vi "Delete Recipe.vi"(8 "error in (no error)":errorcluster, 9 "Delete Row":u16, 11 "Masterv2 in":refnum<class "Masterv2.lvclass">) -> (0 "error out":errorcluster, 3 "Masterv2 out":refnum<class "Masterv2.lvclass">)   [LabVIEW 2014, in "Main Libraryv2.lvlib" / "Masterv2.lvclass"]
uses:
  Master/Masterv2.lvclass
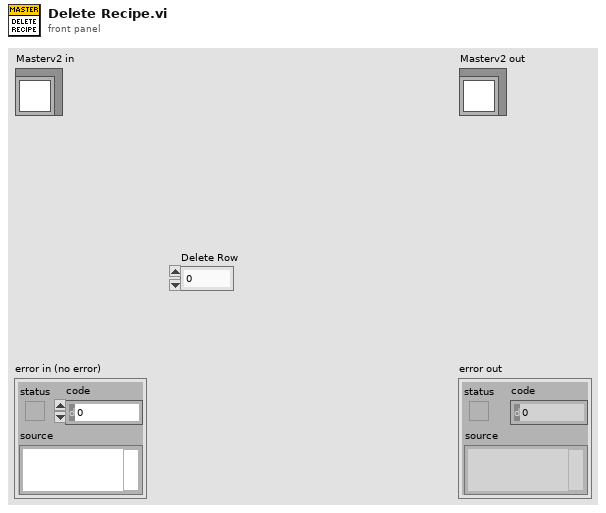
[diagram p1: front panel]
types:
  T1 = cluster{"Speed":string, "Temperature SP":string, "Time Limit":string, "Direction":string}[]
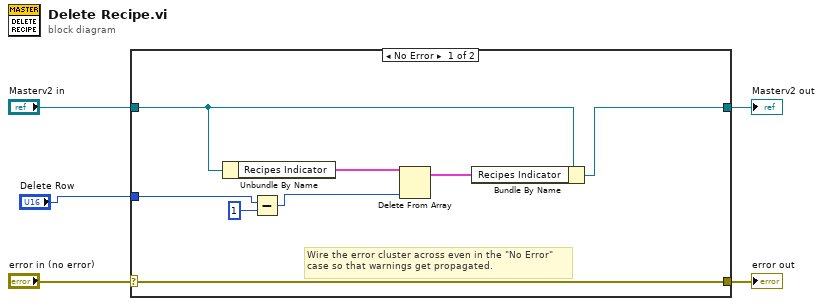
[diagram p0: block diagram]
diagram:
  n1 = case shown="No Error" "error in (no error)" {
    selector: "error in (no error)" -> [w13 w15]
    tunnel: [w13 w15] -> w4
    tunnel: [w6 w14] -> w2
    tunnel: "Masterv2 in" -> [w7 w14]
    tunnel: "Delete Row" -> [w8 _]
    frame No Error {
      # "Wire the error cluster across even in the \"No Error\"\ncase so that warnings get propagated."
      n2 = Unbundle By Name(w7) -> ("Recipes Indicator"=w12:T1)
      n3 = Subtract(x=w8, y=u16 1) -> (x-y=w10:u16)
      n4 = Delete From Array(array=w12, index=w10) -> (array with subset deleted=w11:T1)  [unwired: 1 in, 1 out]
      n5 = Bundle By Name(cluster=w7, "Recipes Indicator"=w11) -> (w6:refnum<class "Masterv2.lvclass">)
    }
    frame Error {
    }
  }
  "error out" <- w4
  "Masterv2 out" <- w2
